vi "Current Position DAO.vi"(7 "Rigid Connection":bool, 8 "LBCB 2 Commands In":dbl[](array[numeric]), 10 "LBCB 1 Commands In":dbl[](array[numeric]), 11 "Actions":T1) -> (0 "LBCB 2 Commands Out":dbl[](array[numeric]), 2 "LBCB 1 Commands Out":dbl[](array[numeric]))   [LabVIEW 2013]
uses:
  Data Access Objects/Metadata/DAO Actions.ctl
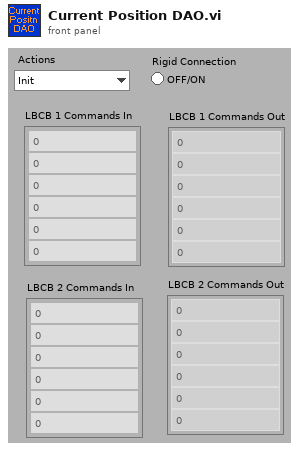
[diagram p1: front panel]
types:
  T1 = typedef "DAO Actions.ctl" = enum16{"Init", "Get", "Set"}
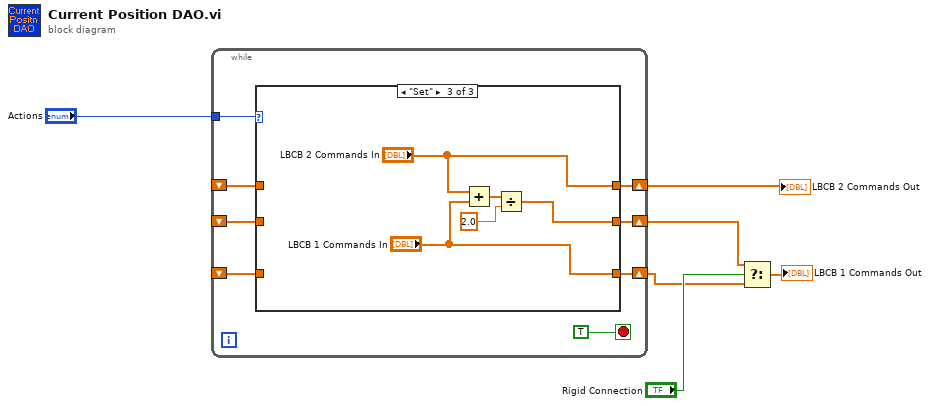
[diagram p0: block diagram]
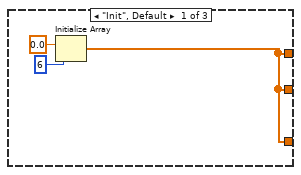
[diagram p2: hidden frame]
diagram:
  n1 = while {
    tunnel: "Actions" -> [w13]
    shift-right: [w12] -> w2
    shift-left: _ -> [w10]
    shift-right: [w11] -> w3
    shift-left: _ -> [w9]
    shift-right: [w8] -> w1
    shift-left: _ -> [w7]
    stop <- TRUE stop-if-true
    n2 = case shown="\"Set\"" w13 {
      tunnel: [w15 w20 "LBCB 1 Commands In"] -> w12
      tunnel: [w15 w19 w21] -> w11
      tunnel: w10 -> [_ w20 _]
      tunnel: w9 -> [_ w19 _]
      tunnel: [w15 w18 "LBCB 2 Commands In"] -> w8
      tunnel: w7 -> [_ w18 _]
      frame "Init", Default {
        n3 = Initialize Array(0.0 ("element"), 6 ("dimension size")) -> (w15:dbl[])
      }
      frame "Get" {
      }
      frame "Set" {
        n4 = Add(x="LBCB 2 Commands In", y="LBCB 1 Commands In") -> (x+y=w23:dbl[])
        n5 = Divide(x=w23, y=2.0) -> (x/y=w21:dbl[])
      }
    }
  }
  "LBCB 2 Commands Out" <- w1
  n6 = Select(t=w3, s="Rigid Connection", f=w2) -> (s? t:f=→"LBCB 1 Commands Out":dbl[])
